vi "UnregisterForDiagPackets.vi"(0 "Event Metadata":T1, 3 "error in (no error)":errorcluster) -> (10 "error out":errorcluster)   [LabVIEW 2010]
uses:
  c:/aerotech/controller/5.xx.xxx/A3200/pc/labview/2010/bin/Aerotech.A3200.LabVIEW.dll
  bin/Aerotech.A3200.LabVIEW.dll
  ControllerDiagPacket.ctl
  AxisDiagPacket.ctl
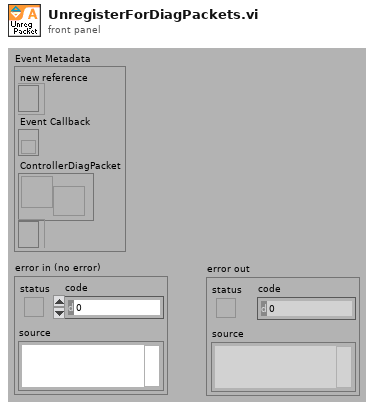
[diagram p1: front panel]
types:
  T1 = cluster{"new reference":refnum<k24>, "Event Callback":refnum<k27>, "ControllerDiagPacket":refnum<user-event>, "Event Registration Refnum 2":refnum<event-registration>}
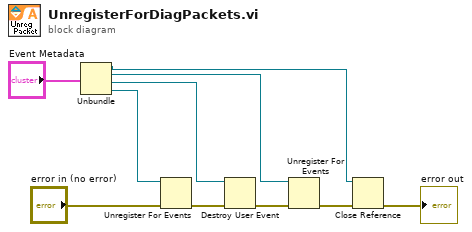
[diagram p0: block diagram]
diagram:
  n1 = Unbundle("Event Metadata") -> ("new reference"=w2:refnum<k24>, "Event Callback"=w3:refnum<k27>, "ControllerDiagPacket"=w4:refnum<user-event>, "Event Registration Refnum 2"=w5:refnum<event-registration>)
  n2 = Unregister For Events(event registration refnum=w5, error in="error in (no error)") -> (error out=w9:errorcluster)
  n3 = Destroy User Event(user event=w4, error in=w9) -> (error out=w8:errorcluster)
  n4 = Unregister For Events(event registration refnum=w3, error in=w8) -> (error out=w7:errorcluster)
  n5 = Close Reference(reference=w2, error in (no error)=w7) -> (error out=→"error out":errorcluster)
